vi "numlock init.vi"(7 "disable buffering? (T)":bool, 8 "error in":errorcluster, 9 "Override file (F)":bool=TRUE, 10 "Default log level (info)":T2(ring)=enum."info", 11 "base path":path) -> (0 "error out":errorcluster, 3 "logger":T1)   [LabVIEW 2019]
doc: "Creates a log file (latest.log.tdms) in the base path specified. If Override file is false, then old files are moved to the format of <date>.tdms"
uses:
  numlock.ctl
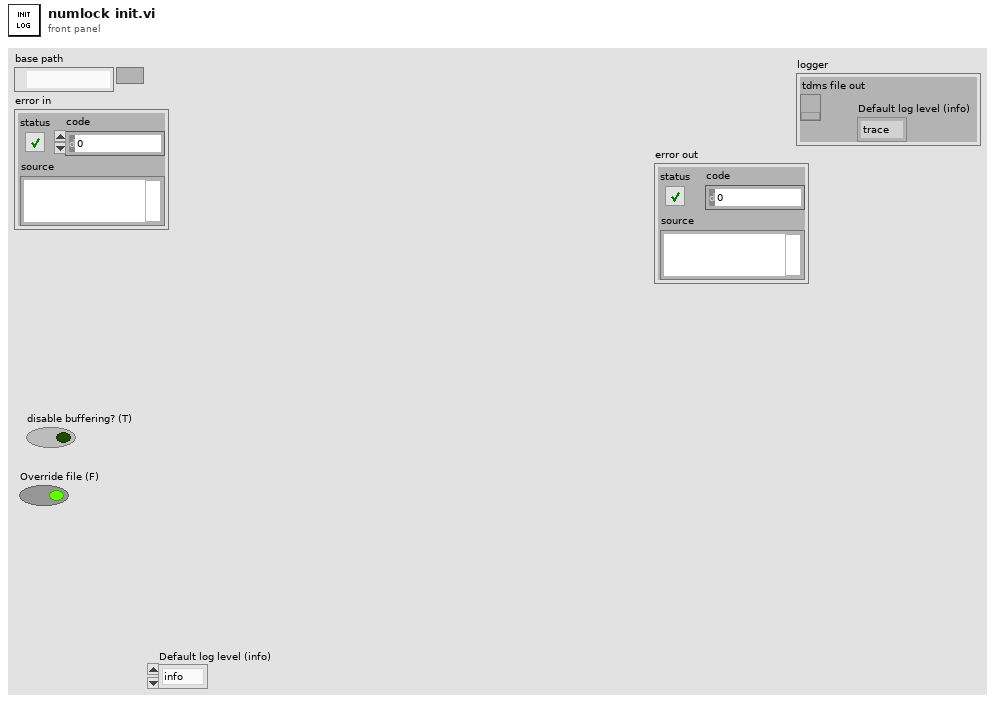
[diagram p1: front panel]
types:
  T1 = typedef "numlock.ctl" = cluster{"tdms file out":refnum<k34>, "Default log level (info)":enum16{"trace", "debug", "info", "warn", "error"}}
  T2 = enum16{"trace", "debug", "info", "warn", "error"}
  T3 = enum16{"open", "open or create", "create or replace", "create", "open (read-only)"}
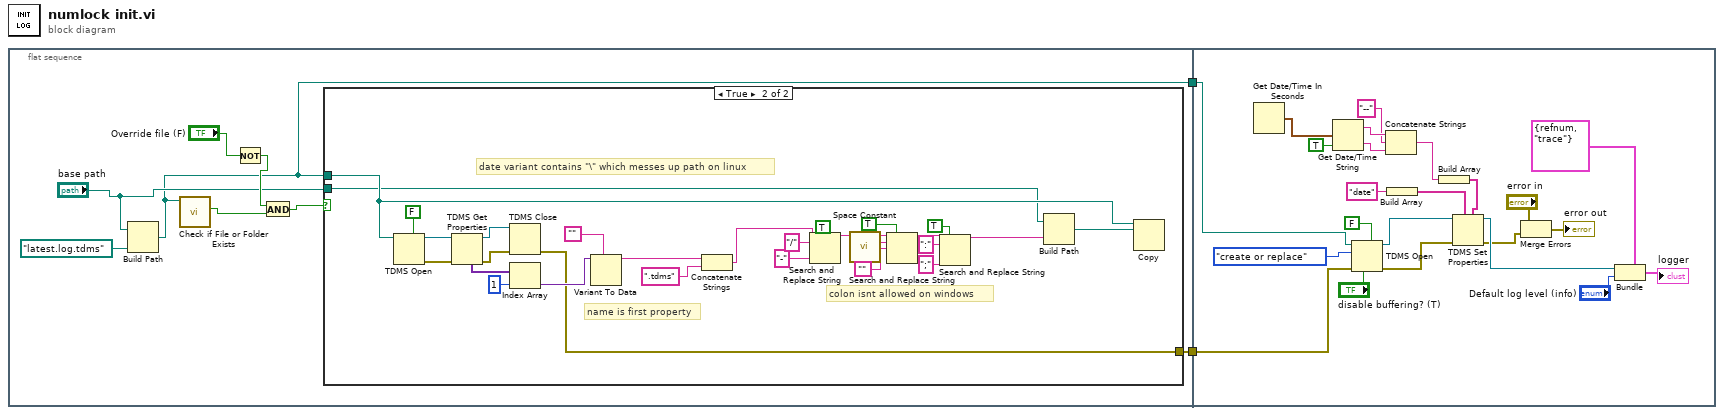
[diagram p0: block diagram]
diagram:
  n1 = flat-sequence {
    tunnel: [w4] -> w2
    tunnel: [w3] -> w1
    tunnel: w2 -> [w51]
    tunnel: w1 -> [w42]
    frame #0 {
      n2 = Build Path(base path="base path", name or relative path=path "latest.log.tdms" ("path")) -> (appended path=w4:path)
      n3 = call <vilib>:"Check if File or Folder Exists.vi"("path"=w4) -> ("file or folder exists?"=w8:bool)  [unwired: 8 in, 2 out]
      n4 = Not(x="Override file (F)") -> (.not. x?=w9:bool)
      n5 = And(x=w9, y=w8) -> (x .and. y?=w10:bool)
      n6 = case shown="True" w10 {
        tunnel: w4 -> [_ w30]
        tunnel: "base path" -> [_ w28]
        tunnel: [_ w11] -> w3
        frame False {
        }
        frame True {
          # "colon isnt allowed on windows"
          # "date variant contains \"\\\" which messes up path on linux"
          # "name is first property"
          n7 = TDMS Open(5:FALSE ("create index file? (T)"), 11:w30) -> (0:w13:errorcluster, 3:w37:refnum<k34>)  [unwired: 5 in]
          n8 = TDMS Get Properties(8:w13, 11:w37) -> (0:w12:errorcluster, 3:w19:refnum<k34>, 4:w36:variant[])  [unwired: 4 in, 3 out]
          n9 = TDMS Close(8:w12, 11:w19) -> (0:w11:errorcluster)  [unwired: 1 out]
          n10 = Index Array(array=w36, index=1) -> (element=w34:variant)
          n11 = Variant To Data(type="", Variant=w34) -> (data=w31:string)  [unwired: 1 in, 1 out]
          n12 = Concatenate Strings(w31, ".tdms" ("string")) -> (w27:string)
          n13 = Search and Replace String(replace all?=TRUE ("replace all? (F)"), input string=w27, search string="/", replace string="-" ("replace string (\"\")")) -> (result string=w23:string)  [unwired: 4 in, 3 out]
          n14 = call <vilib>:"Space Constant.vi"() -> ("String"=w22:string)
          n15 = Search and Replace String(replace all?=TRUE ("replace all? (F)"), input string=w23, search string=w22, replace string="") -> (result string=w18:string)  [unwired: 4 in, 3 out]
          n16 = Search and Replace String(replace all?=TRUE ("replace all? (F)"), input string=w18, search string=":", replace string=";" ("replace string (\"\")")) -> (result string=w17:string)  [unwired: 4 in, 3 out]
          n17 = Build Path(base path=w28, name or relative path=w17) -> (appended path=w29:path)
          n18 = Copy(10:w29, 11:w30) -> ()  [unwired: 3 in, 3 out]
        }
      }
    }
    frame #1 {
      n19 = Get Date/Time In Seconds() -> (seconds since 1Jan1904=w50:timestamp)
      n20 = Get Date/Time String(seconds (now)=w50, want seconds? (F)=TRUE) -> (date string=w49:string, time string=w47:string)  [unwired: 1 in]
      n21 = TDMS Open(5:FALSE ("create index file? (T)"), 6:"disable buffering? (T)", 8:w42, 10:T3."create or replace" ("operation (0:open)"), 11:w51) -> (0:w43:errorcluster, 3:w60:refnum<k34>)  [unwired: 2 in]
      n22 = Concatenate Strings(w49, "--" ("string"), w47) -> (w46:string)
      n23 = Build Array("date") -> (w54:string[])
      n24 = Build Array(w46) -> (w45:string[])
      n25 = TDMS Set Properties(5:w45, 7:w54, 8:w43, 11:w60) -> (0:w41:errorcluster, 3:w61:refnum<k34>)  [unwired: 2 in, 2 out]
      n26 = Merge Errors("error in", w41) -> (→"error out":errorcluster)
      n27 = Bundle(cluster=T1 {"tdms file out"=refnum, "Default log level (info)"=enum."trace"} ("logger"), "tdms file out"=w61, "Default log level (info)"="Default log level (info)") -> (→"logger":T1)
    }
  }
